vi "Set Number of Dimensions.vi"(10 "No. of Dimensions (1)":u32=1, 11 "Array Writer in":refnum<class "Array Writer.lvclass">) -> (3 "Array Writer out":refnum<class "Array Writer.lvclass">)   [LabVIEW 2013, in "Array Writer.lvclass"]
doc: "Copyright (c) 2016 Sze Howe Koh\n\nThis Source Code Form is subject to the terms of the Mozilla Public License, v. 2.0. If a copy of the MPL was not distributed with this file, You can obtain one at http://mozilla.org/MPL/2.0/."
uses:
  Array Writer.lvclass
  Array Writer.lvclass/Array Writer.ctl
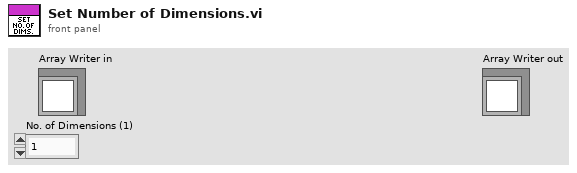
[diagram p1: front panel]
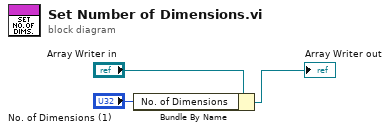
[diagram p0: block diagram]
diagram:
  n1 = Bundle By Name(cluster="Array Writer in", "No. of Dimensions"="No. of Dimensions (1)") -> (→"Array Writer out":refnum<class "Array Writer.lvclass">)
